vi "RenderDiff.vi"(8 "error in (no error)":errorcluster, 9 "-OutputDir":path, 10 "-PathToNewVI":path, 11 "-PathToOldVI":path) -> (0 "error out":errorcluster)   [LabVIEW 2020, in "CICD.lvlib"]
uses:
  CICD.lvlib
  Diff/Screenshots/VIDiffScreenshots.lvlib
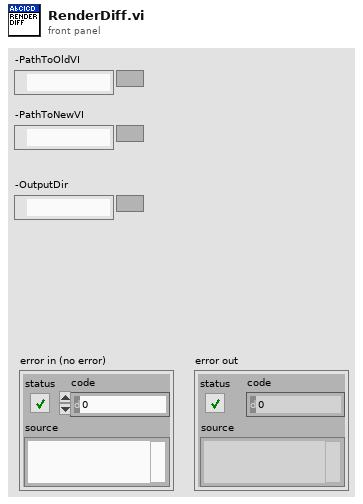
[diagram p1: front panel]
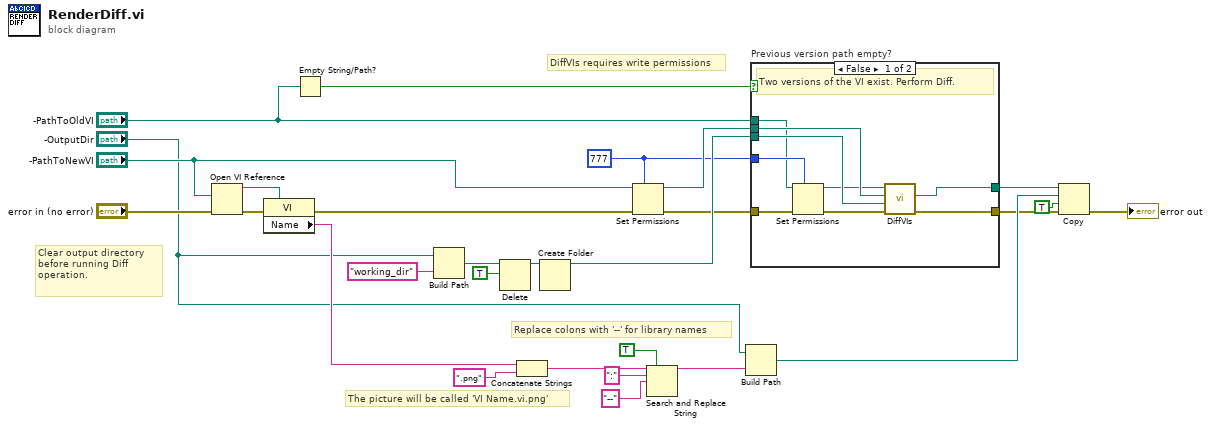
[diagram p0: block diagram]
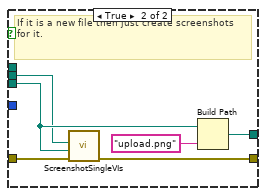
[diagram p2: hidden frame]
diagram:
  w1 = i16 777 ("permissions")
  # "Replace colons with '--' for library names"
  # "Clear output directory before running Diff operation."
  # "DiffVIs requires write permissions"
  # "The picture will be called 'VI Name.vi.png'"
  n1 = Open VI Reference(vi path="-PathToNewVI", error in (no error)="error in (no error)") -> (vi reference=w18:refnum<vi>, error out=w19:errorcluster)  [unwired: 4 in]
  n2 = property class="VI"(reference=w18, error in=w19) -> (error out=w2:errorcluster, "Name"=w20:string)  [unwired: 1 out]
  n3 = Empty String/Path?(string/path="-PathToOldVI") -> (empty?=w8:bool)
  n4 = Build Path(base path="-OutputDir", name or relative path="working_dir") -> (appended path=w21:path)
  n5 = Delete(path (use dialog)=w21, entire hierarchy (F)=TRUE) -> (deleted path=w22:path)  [unwired: 3 in, 2 out]
  n6 = Concatenate Strings(w20, ".png" ("string")) -> (w27:string)
  n7 = Create Folder(path (use dialog)=w22) -> (created path=w12:path)  [unwired: 2 in, 2 out]
  n8 = Set Permissions(7:w1, 8:w2, 11:"-PathToNewVI") -> (0:w9:errorcluster, 3:w10:path)  [unwired: 2 in]
  n9 = Search and Replace String(replace all?=TRUE ("replace all? (F)"), input string=w27, search string=":", replace string="--" ("replace string (\"\")")) -> (result string=w24:string)  [unwired: 4 in, 3 out]
  n10 = Build Path(base path="-OutputDir", name or relative path=w24) -> (appended path=w16:path)
  n11 = case "Previous version path empty?" shown="False" w8 {
    tunnel: w9 -> [w32 w39]
    tunnel: w10 -> [w37 w38]
    tunnel: [w36 w43] -> w11
    tunnel: w12 -> [w35 w40]
    tunnel: [w34 w41] -> w13
    tunnel: "-PathToOldVI" -> [w30 _]
    tunnel: w1 -> [w31 _]
    frame False {
      # "Two versions of the VI exist. Perform Diff."
      n12 = Set Permissions(7:w31, 8:w32, 11:w30) -> (0:w33:errorcluster, 3:w29:path)  [unwired: 2 in]
      n13 = call "DiffVIs.vi"("error in"=w33, "Picture Save Location"=w35, "New VI Path"=w37, "Old VI Path"=w29) -> ("error out"=w34:errorcluster, "diff file"=w36:path)  [unwired: 6 in]
    }
    frame True {
      # "If it is a new file then just create screenshots for it."
      n14 = call "ScreenshotSingleVIs.vi"("error in"=w39, "Picture Save Location"=w40, "New VI Path"=w38) -> ("error out"=w41:errorcluster)  [unwired: 8 in]
      n15 = Build Path(base path=w40, name or relative path="upload.png") -> (appended path=w43:path)
    }
  }
  n16 = Copy(8:w13, 9:TRUE ("overwrite (F)"), 10:w16, 11:w11) -> (0:→"error out":errorcluster)  [unwired: 1 in, 2 out]
